vi "C.vi"(10 "6":string[](array[string]), 11 "CF":string) -> (3 "C":string)   [LabVIEW 2017]
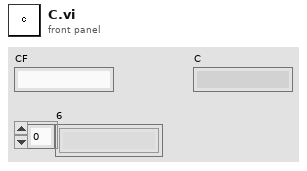
[diagram p1: front panel]
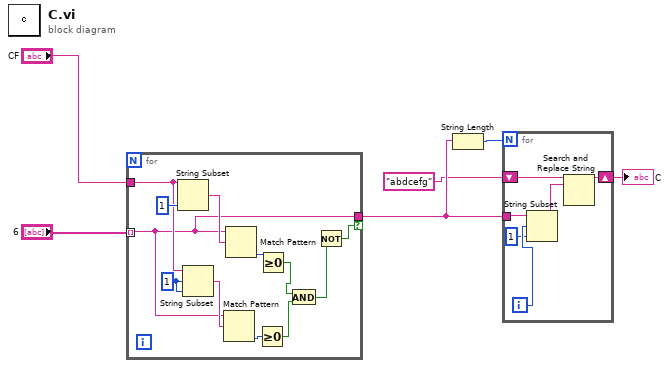
[diagram p0: block diagram]
diagram:
  n1 = for {
    tunnel: "6" -> [w8] mode=indexing
    tunnel: "CF" -> [w16]
    tunnel: [w8] -> w5 if=w7
    w15 = 1 ("offset (0)")
    n2 = String Subset(string=w16, length (rest)=1 ("length (rest)")) -> (substring=w17:string)  [unwired: 1 in]
    n3 = String Subset(string=w16, offset (0)=w15, length (rest)=w15) -> (substring=w14:string)
    n4 = Match Pattern(string=w8, regular expression=w14) -> (offset past match=w12:i32)  [unwired: 1 in, 3 out]
    n5 = Match Pattern(string=w8, regular expression=w17) -> (offset past match=w13:i32)  [unwired: 1 in, 3 out]
    n6 = Greater Or Equal To 0?(x=w12) -> (x >= 0?=w10:bool)
    n7 = Greater Or Equal To 0?(x=w13) -> (x >= 0?=w11:bool)
    n8 = And(x=w11, y=w10) -> (x .and. y?=w9:bool)
    n9 = Not(x=w9) -> (.not. x?=w7:bool)
  }
  n10 = String Length(string=w5) -> (length=w3:i32)
  n11 = for {
    N: w3 -> [_]
    tunnel: w5 -> [w22]
    shift-right: [w23] -> w6
    shift-left: "abdcefg" -> [w24]
    i -> [w20]
    n12 = String Subset(string=w22, offset (0)=w20, length (rest)=1 ("length (rest)")) -> (substring=w21:string)
    n13 = Search and Replace String(input string=w24, search string=w21) -> (result string=w23:string)  [unwired: 6 in, 3 out]
  }
  "C" <- w6
